vi "Main.vi"(11 "Module Admin":refnum<class "Delacor_lib_QMH_Module Admin.lvclass">) -> ()   [LabVIEW 2021, in "RT-TDMS-Logging.lvlib"]
doc: "This template is based off of the Queued Message Handler design pattern and the Queued Message Handler project template that ships with LabVIEW.\n\nThe main difference is that the queue is private to this module and communication between modules is performed via Broadcast and Request events.\n\nRequest events are wrapped in public API methods and are handled in the Event Handling Loop (EHL) of this VI. Any module can register for Broadcast events sent by this module. The EHL generates messages based on user interface actions.\n\nThe Message Handling Loop (MHL) processes messages generated by the EHL, or by other messages. The messages are string values, so new messages can be added easily to the Message Cases case structure in the MHL. Each message cluster can also provide an optional value for Message Data, which is a variant that can be converted to whatever message-specific data is required.\n_____\nBased on DQMH Project Template 7.0.1.1316."
uses:
  RT-TDMS-Logging.lvlib
  <vilib>/Delacor/Delacor QMH/Libraries/Module Admin_class/Delacor_lib_QMH_Module Admin.lvclass
  Module Data--cluster.ctl
  <vilib>/Wovalab/Utilities/Helper Loop Periodic Timing/Helper Loop Periodic Timing.lvclass/Helper Loop Periodic Timing.ctl
  <vilib>/Delacor/Delacor QMH/Libraries/Message Queue_class/Delacor_lib_QMH_Message Queue.lvclass/Delacor_lib_QMH_Message Queue.ctl
  Start Logging Argument--cluster.ctl
  Data Logging Duration Argument--cluster.ctl
  Stop Argument--cluster.ctl
  <vilib>/Delacor/Delacor QMH/Libraries/Module Admin_class/Delacor_lib_QMH_Module Admin.lvclass/Delacor_lib_QMH_Module Admin.ctl
  AI Data's Argument--cluster.ctl
  DO Data Argument--cluster.ctl
  <vilib>/Utility/miscctls.llb/LVPointTypeDef.ctl
  Main Engine/Controls/Main Engine Q Option.ctl
  Host-Control's/TCP Tx-Rx cluster.ctl
  <vilib>/Delacor/Delacor QMH/Libraries/Message Queue_class/Delacor_lib_QMH_Enqueue Message (Single).vi
  <vilib>/Delacor/Delacor QMH/Libraries/Module Admin_class/Delacor_lib_QMH_Get External Launch.vi
  <vilib>/Wovalab/Utilities/Helper Loop Periodic Timing/U32 Max Value--constant.vi
  <vilib>/Wovalab/Utilities/Helper Loop Periodic Timing/Update Last Execution Time.vi
  <vilib>/Wovalab/Utilities/Helper Loop Periodic Timing/Helper Loop Periodic Timing.lvclass
  <vilib>/Delacor/Delacor QMH/Libraries/Message Queue_class/Delacor_lib_QMH_Message Queue.lvclass
  <vilib>/addons/_JKI.lib/Serialization/JSON/JKI JSON Serialization.lvlib
panel:
  out "error out":errorcluster
  out "Status":string
  in  "Simulate MHL Error":bool
  in  "Simulate EHL Error":bool
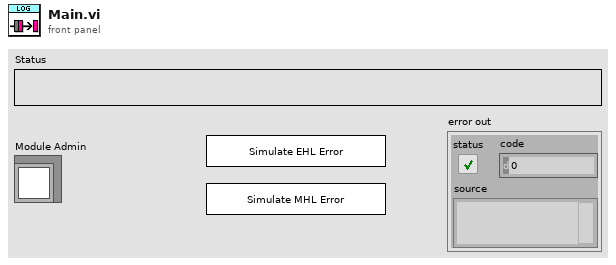
[diagram p1: front panel]
types:
  T1 = typedef "RT-TDMS-Logging.lvlib/Request Events--cluster.ctl" = cluster{"Stop Module":refnum<user-event>, "Show Panel":refnum<user-event>, "Hide Panel":refnum<user-event>, "Get Module Execution Status":refnum<user-event>, "Show Diagram":refnum<user-event>, "Data Logging Duration":refnum<user-event>, "AI Data's":refnum<user-event>, "Start Logging":refnum<user-event>, "DO Data":refnum<user-event>}
  T2 = typedef "RT-TDMS-Logging.lvlib/Start Logging Argument--cluster.ctl" = cluster{"Start Logging":variant}
  T3 = enum32{"invalid lock state", "Not Locked", "Locked (No Password)", "Password-protected"}
  T4 = typedef "RT-TDMS-Logging.lvlib/Stop Argument--cluster.ctl" = cluster{"Origin":string, "Exit via Stop Module Req?":bool, "Wait for Module to stop?":bool}
  T5 = typedef "RT-TDMS-Logging.lvlib/AI Data's Argument--cluster.ctl" = cluster{"AI Data's":variant}
  T6 = typedef "RT-TDMS-Logging.lvlib/DO Data Argument--cluster.ctl" = cluster{"DO Data":variant}
  T7 = typedef "LVPointTypeDef.ctl" = cluster{"Horizontal":i16, "Vertical":i16}
  T8 = enum32{"Invalid", "Standard", "Closed", "Hidden", "Minimized", "Maximized"}
  T9 = typedef "Main Engine Q Option.ctl" = enum16{"Init", "Get"}
  T10 = cluster{"Time Stamp":timestamp[], "Identification Names":string[], "Data":dbl[]}
  T11 = cluster{"Identification Name":string[], "Data":i16[]}
  T12 = enum16{"open", "open or create", "create or replace", "create", "open (read-only)"}
  T13 = typedef "TCP Tx-Rx cluster.ctl" = cluster{"Interface":string, "Command":string, "SubCmd":string, "Data":variant}
  T14 = typedef "RT-TDMS-Logging.lvlib/Module Data--cluster.ctl" = cluster{"Status":string, "TDMS-Folder":path, "Data Logging Time (S)":dbl, "Start -Log":bool, "Stop -Log":bool, "tdms file out":refnum<k34>, "Start Time":timestamp, "Interface Data's":cluster{"AO Data's":map{string, dbl}, "DI Data's":map{string, i16}, "DO Data's":map{string, i16}, "AI Data's":map{string, waveform(dbl)}}, "TCP Enigine Q":refnum<queue>}
  T15 = typedef "RT-TDMS-Logging.lvlib/Data Logging Duration Argument--cluster.ctl" = cluster{"Data Logging Duration(Sec)":dbl}
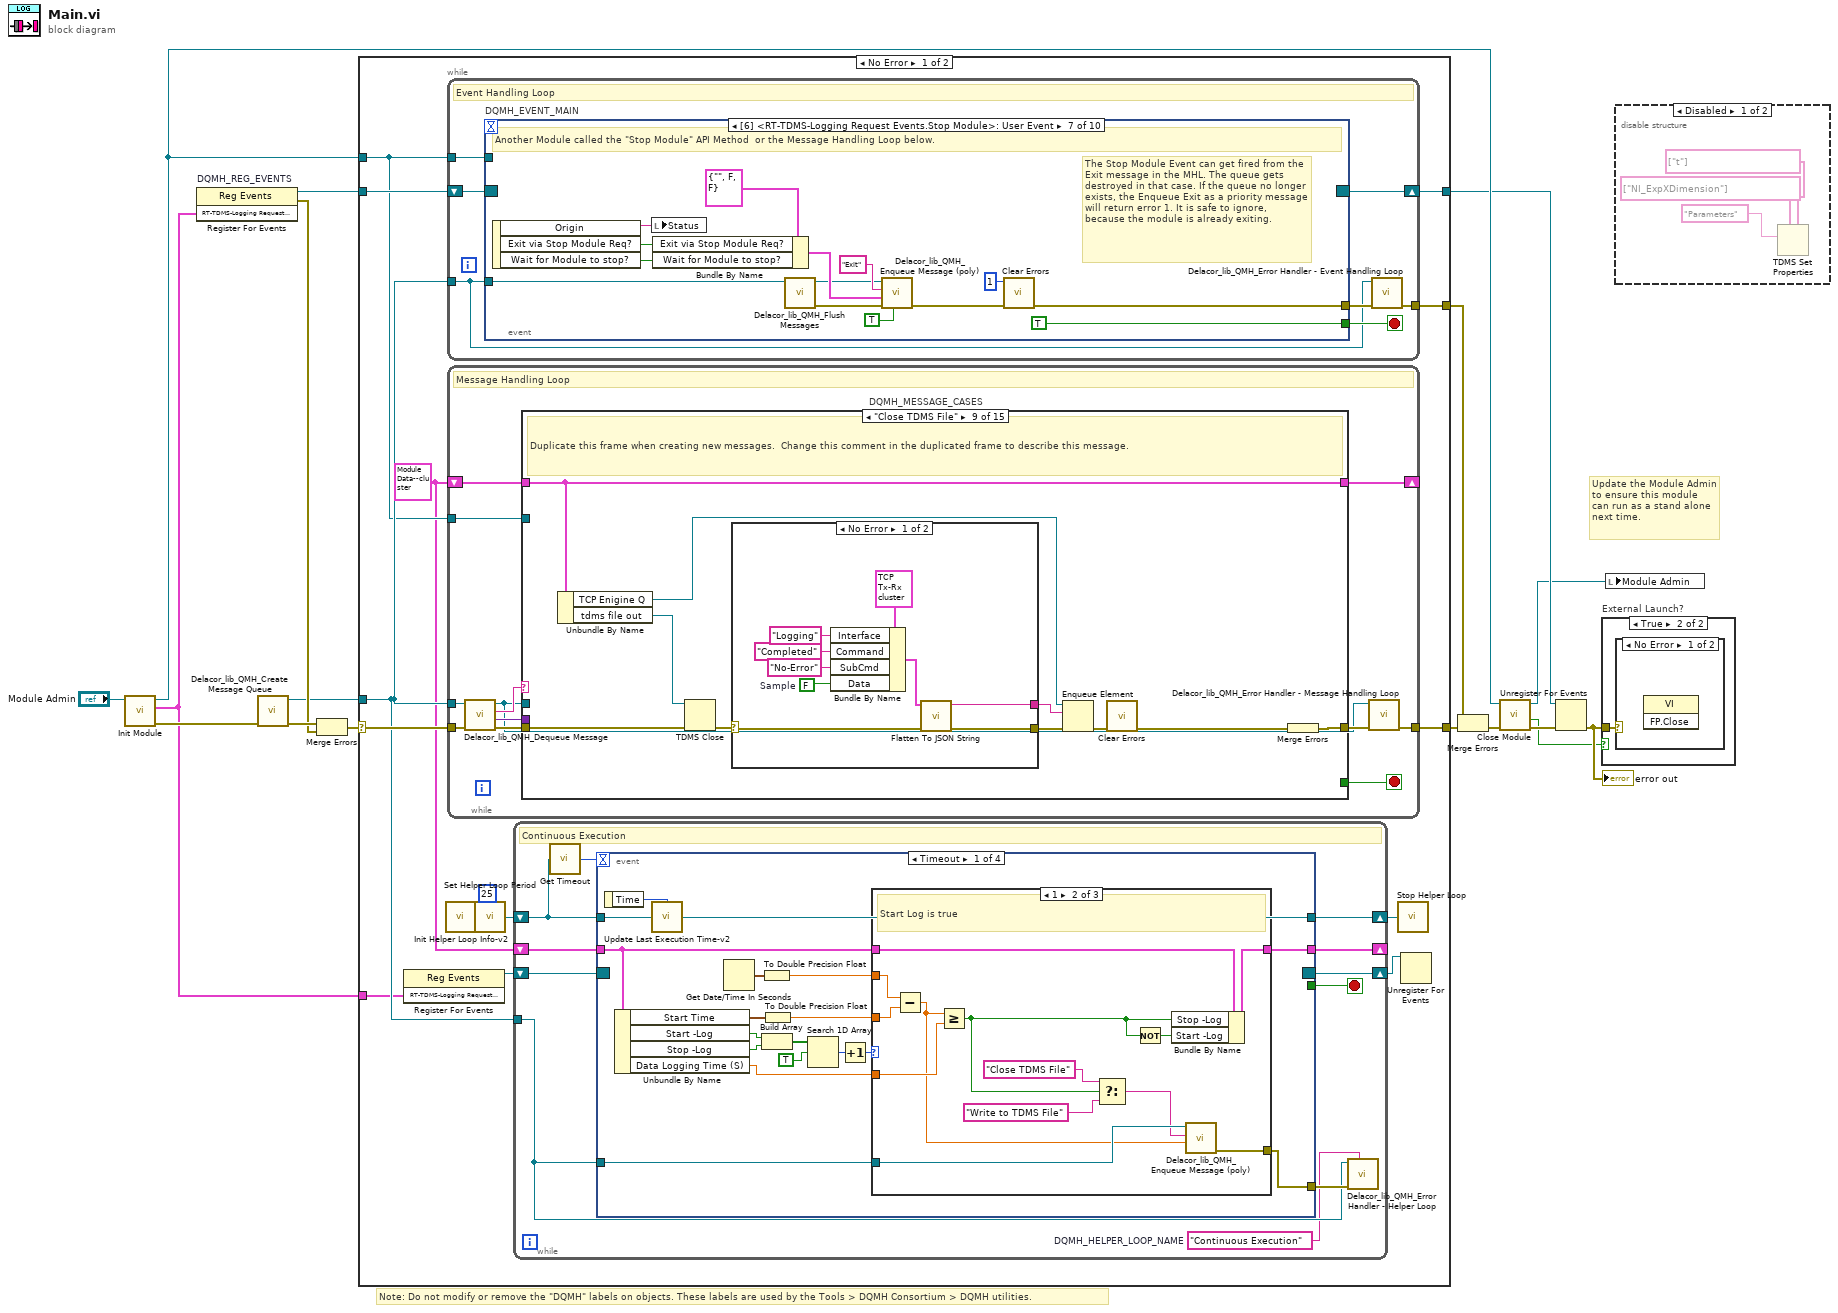
[diagram p0: block diagram]
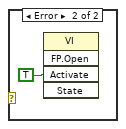
[diagram p4: hidden frame]
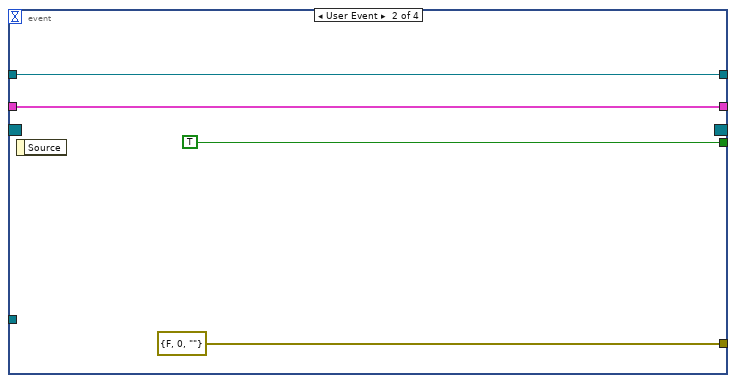
[diagram p7: hidden frame]
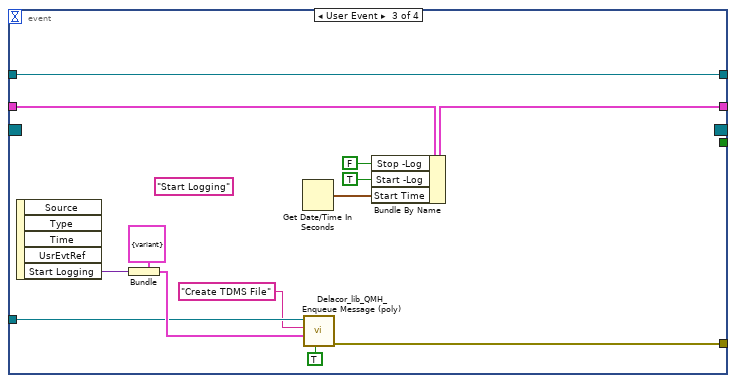
[diagram p8: hidden frame]
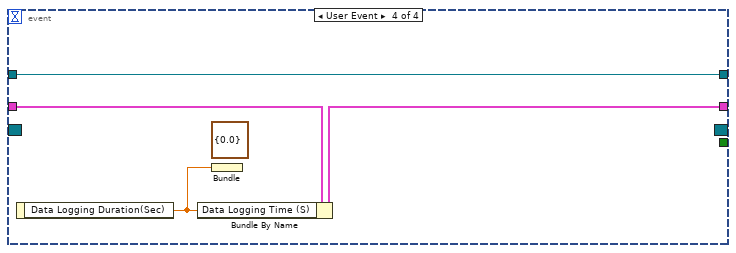
[diagram p9: hidden frame]
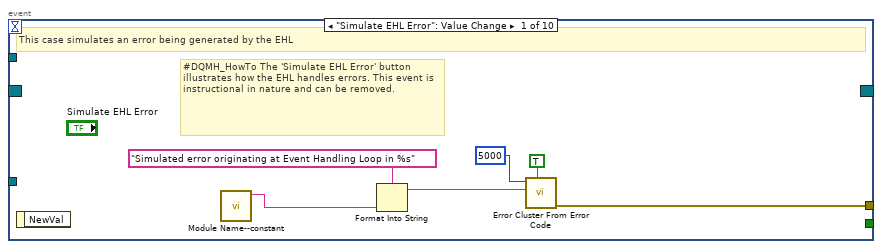
[diagram p10: hidden frame]
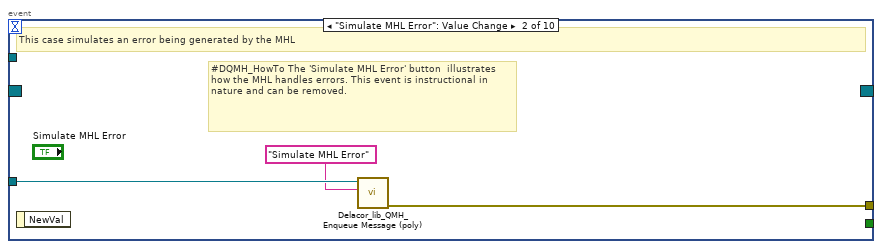
[diagram p11: hidden frame]
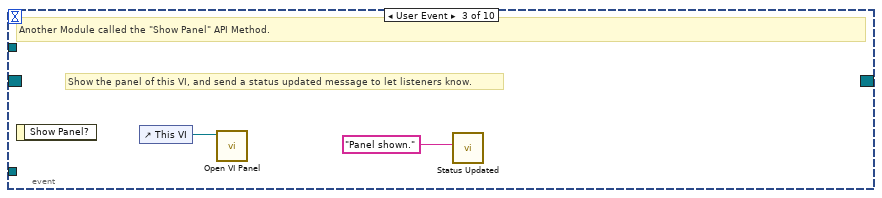
[diagram p12: hidden frame]
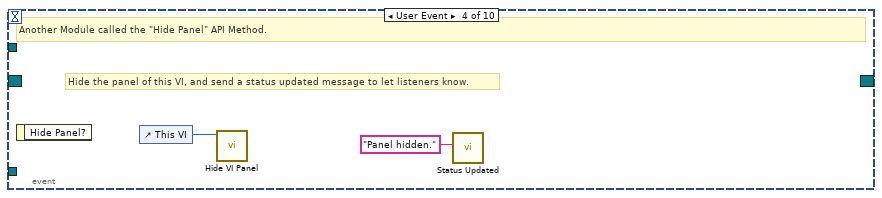
[diagram p13: hidden frame]
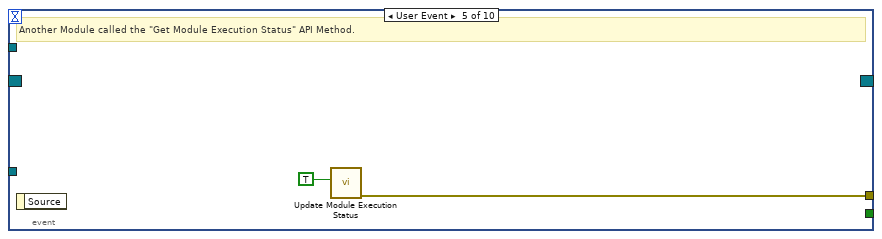
[diagram p14: hidden frame]
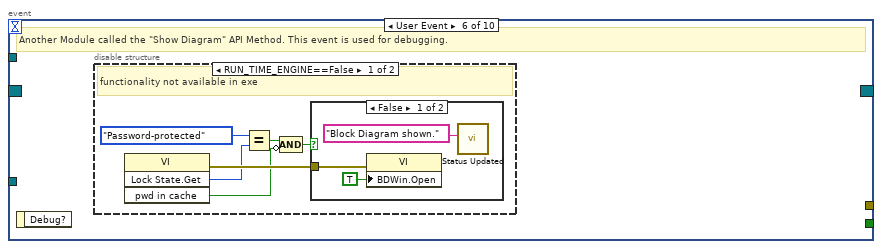
[diagram p15: hidden frame]
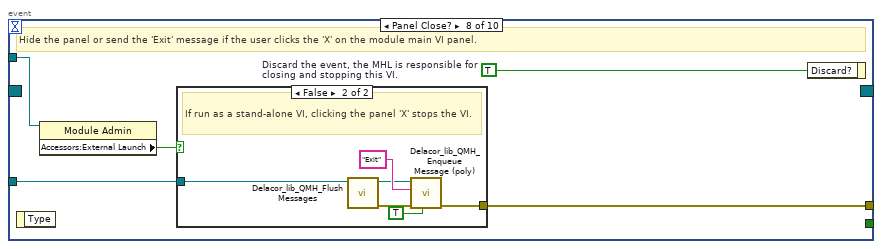
[diagram p18: hidden frame]
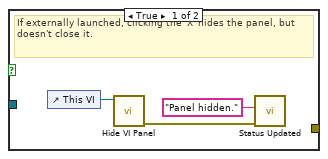
[diagram p19: hidden frame]
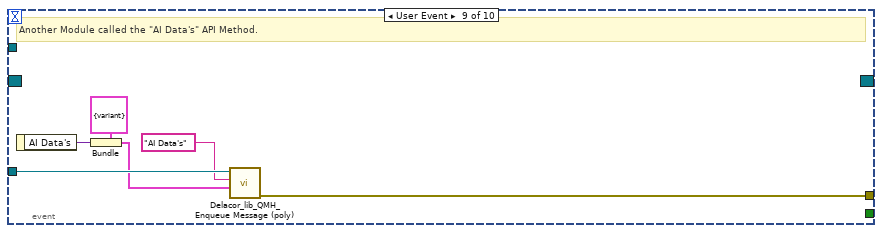
[diagram p20: hidden frame]
diagram:
  # "Note: Do not modify or remove the \"DQMH\" labels on objects. These labels are used by the Tools > DQMH Consortium > DQMH utilities."
  # "Update the Module Admin to ensure this module can run as a stand alone next time."
  n1 = call "Init Module.vi"("Singleton Module Admin in"="Module Admin") -> ("error out"=w16:errorcluster, "RT-TDMS-Logging Request Events"=w1:T1, "Singleton Module Admin out"=w8:refnum<class "Delacor_lib_QMH_Module Admin.lvclass">)  [unwired: 8 in]
  n2 = register-events "DQMH_REG_EVENTS"(w1) -> (reference out=w6:refnum<event-registration>, error out=w9:errorcluster)  [unwired: 2 in]
  n3 = call <vilib>:"Delacor_lib_QMH_Create Message Queue.vi"("error in"=w16) -> ("error out"=w11:errorcluster, "Message Queue"=w5:refnum<class "Delacor_lib_QMH_Message Queue.lvclass">)  [unwired: 9 in]
  n4 = Merge Errors(w11, w9) -> (w10:errorcluster)
  n5 = case shown="No Error" w10 {
    selector: w10 -> [w30 w438]
    tunnel: [w32 w437] -> w17
    tunnel: [w29 w436] -> w7
    tunnel: w6 -> [w28 w436]
    tunnel: w5 -> [w27 w431]
    tunnel: [w31 _] -> w14
    tunnel: w8 -> [w26 w432]
    tunnel: w1 -> [w25 _]
    frame No Error {
      w18 = T14 {"Status"="", "TDMS-Folder"=path "", "Data Logging Time (S)"=0.0, "Start -Log"=FALSE, "Stop -Log"=FALSE, "tdms file out"=refnum, "Start Time"=timestamp(0 s since 1904-01-01), "Interface Data's"={"AO Data's"={}, "DI Data's"={}, "DO Data's"={}, "AI Data's"={}}, "TCP Enigine Q"=refnum} ("Data Cluster")
      n6 = register-events ("DQMH_HELPER_REGFOREVENTS")(w25) -> (reference out=w23:refnum<event-registration>)  [unwired: 2 in, 1 out]
      n7 = call <vilib>:"Init Helper Loop Info-v2.vi"() -> ("Helper Loop Periodic Timing"=w21:refnum<class "Helper Loop Periodic Timing.lvclass">)  [unwired: 1 in]
      n8 = while {
        tunnel: w27 -> [w98]
        shift-right: [w101] -> w29
        shift-left: w28 -> [w102]
        tunnel: [w103] -> w31
        tunnel: w26 -> [w99]
        stop <- w100 stop-if-true
        # "Event Handling Loop"
        n9 = event "DQMH_EVENT_MAIN" shown="[6] <RT-TDMS-Logging Request Events.Stop Module>: User Event" {
          selector: w102 -> [_ _ _ _ _ _ _ _ _ _]
          dyn-events: [_ _ _ _ _ _ _ _ _ _] -> w101
          timeout: _ -> [_ _ _ _ _ _ _ _ _ _]
          tunnel: [_ _ _ _ _ _ TRUE ("Discard?") _ _ _] -> w100
          tunnel: w98 -> [_ w112 _ _ _ _ w131 w145 w162 w168]
          tunnel: [w110 w113 _ _ w119 _ w141 w147 w157 w163] -> w104
          tunnel: w99 -> [_ _ _ _ _ _ _ w144 _ _]
          event "Simulate EHL Error": Value Change {
            # "#DQMH_HowTo The 'Simulate EHL Error' button  illustrates how the EHL handles errors. This event is instructional in nature and can be removed."
            # "This case simulates an error being generated by the EHL"
            n10 = event-data() -> ()  [unwired: 1 in, 1 out]
            n11 = call "Module Name--constant.vi"() -> ("Module Name"=w107:string)  [unwired: 11 in]
            n12 = Format Into String(format string="Simulated error originating at Event Handling Loop in %s", w107) -> (resulting string=w108:string)  [unwired: 2 in, 1 out]
            n13 = call <vilib>:"Error Cluster From Error Code.vi"("show call chain? (False)"=TRUE, "error message (\"\")"=w108, "error code (0)"=5000) -> ("error out"=w110:errorcluster)  [unwired: 6 in]
          }
          event "Simulate MHL Error": Value Change {
            # "#DQMH_HowTo The 'Simulate MHL Error' button  illustrates how the MHL handles errors. This event is instructional in nature and can be removed."
            # "This case simulates an error being generated by the MHL"
            n14 = event-data() -> ()  [unwired: 1 in, 1 out]
            n15 = call-poly <vilib>:"Delacor_lib_QMH_Enqueue Message (poly).vi"("Message"="Simulate MHL Error", "Message Queue in"=w112) -> ("error out"=w113:errorcluster)  [unwired: 8 in, 1 out]
          }
          event User Event {
            # "Show the panel of this VI, and send a status updated message to let listeners know."
            # "Another Module called the \"Show Panel\" API Method."
            n16 = event-data() -> ()  [unwired: 1 in, 1 out]
            n17 = control-ref of="This VI"() -> (w115:refnum<vi>)
            n18 = call "Open VI Panel.vi"("VI"=w115) -> ()  [unwired: 10 in, 1 out]
            n19 = call "Status Updated.vi"("Status"="Panel shown." ("format string")) -> ()  [unwired: 10 in, 1 out]
          }
          event User Event {
            # "Hide the panel of this VI, and send a status updated message to let listeners know."
            # "Another Module called the \"Hide Panel\" API Method."
            n20 = event-data() -> ()  [unwired: 1 in, 1 out]
            n21 = control-ref of="This VI"() -> (w117:refnum<vi>)
            n22 = call "Hide VI Panel.vi"("VI"=w117) -> ()  [unwired: 10 in, 1 out]
            n23 = call "Status Updated.vi"("Status"="Panel hidden." ("format string")) -> ()  [unwired: 10 in, 1 out]
          }
          event User Event {
            # "Another Module called the \"Get Module Execution Status\" API Method."
            n24 = event-data() -> ()  [unwired: 1 in, 1 out]
            n25 = call "Update Module Execution Status.vi"("Running?"=TRUE) -> ("error out"=w119:errorcluster)  [unwired: 10 in]
          }
          event User Event {
            # "Another Module called the \"Show Diagram\" API Method. This event is used for debugging."
            n26 = event-data() -> ()  [unwired: 1 in, 1 out]
            n27 = disable-structure shown="RUN_TIME_ENGINE==False" {
              frame condition #0 (active) {
                # "functionality not available in exe"
                n28 = invoke on="Invoke Node" class="VI" method="Lock State.Get"() -> (error out=w125:errorcluster, "Get Lock State"=w124:T3, "pwd in cache"=w121:bool)  [unwired: 4 in, 1 out]
                n29 = Equal?(x=T3."Password-protected", y=w124) -> (x = y?=w122:bool)
                n30 = Compound Arithmetic op=AND(w122, invert w121) -> (w120:bool)
                n31 = case shown="False" w120 {
                  tunnel: w125 -> [w128 _]
                  frame False {
                    n32 = property on="Property Node" class="VI"(error in=w128, "BDWin.Open"=TRUE ("Block Diagram Window:Open")) -> ()  [unwired: 1 in, 2 out]
                    n33 = call "Status Updated.vi"("Status"="Block Diagram shown." ("format string")) -> ()  [unwired: 10 in, 1 out]
                  }
                  frame True {
                    # "Password-protected VI, and the password is not in the cache. Do not show the diagram."
                  }
                }
              }
              frame condition #1 {
              }
            }
          }
          event User Event {
            # "The Stop Module Event can get fired from the Exit message in the MHL. The queue gets destroyed in that case. If the queue no longer exists, the Enqueue Exit as a priority message will return error 1. It is safe to ignore, because the module is already exiting."
            # "Another Module called the \"Stop Module\" API Method  or the Message Handling Loop below."
            n34 = event-data() -> ("Origin"=w138:string, "Exit via Stop Module Req?"=w134:bool, "Wait for Module to stop?"=w133:bool)  [unwired: 1 in]
            n35 = local write "Status"(w138) -> ()
            n36 = Bundle By Name(cluster=T4 {"Origin"="", "Exit via Stop Module Req?"=FALSE, "Wait for Module to stop?"=FALSE} ("Stop Argument"), "Exit via Stop Module Req?"=w134, "Wait for Module to stop?"=w133) -> (w132:T4)
            n37 = call-dynamic "Delacor_lib_QMH_Flush Messages.vi"("Message Queue in"=w131) -> ("error out"=w129:errorcluster, "Message Queue out"=w130:refnum<class "Delacor_lib_QMH_Message Queue.lvclass">)  [unwired: 7 in, 2 out]
            n38 = call-poly <vilib>:"Delacor_lib_QMH_Enqueue Message (poly).vi"("Priority Message? (F)"=TRUE, "error in"=w129, "Message Data"=w132, "Message"="Exit", "Message Queue in"=w130) -> ("error out"=w142:errorcluster)  [unwired: 5 in, 1 out]
            n39 = call <vilib>:"Clear Errors.vi"("error in (no error)"=w142, "specific error code to clear (0: all)"=1) -> ("error out"=w141:errorcluster)  [unwired: 4 in, 1 out]
          }
          event Panel Close? {
            w146 = TRUE  # Discard the event, the MHL is responsible for closing and stopping this VI.
            # "Hide the panel or send the 'Exit' message if the user clicks the 'X' on the module main VI panel."
            n40 = event-data() -> ()  [unwired: 1 in, 1 out]
            n41 = property on="Property Node" class="Module Admin"(reference=w144) -> ("Accessors:External Launch"=w143:bool)  [unwired: 1 in, 2 out]
            n42 = case shown="False" w143 {
              tunnel: w145 -> [_ w153]
              tunnel: [_ w156] -> w147
              frame True {
                # "If externally launched, clicking the 'X' hides the panel, but doesn't close it."
                n43 = control-ref of="This VI"() -> (w150:refnum<vi>)
                n44 = call "Hide VI Panel.vi"("VI"=w150) -> ("error out"=w148:errorcluster)  [unwired: 10 in]
                n45 = call "Status Updated.vi"("error in"=w148, "Status"="Panel hidden." ("format string")) -> ()  [unwired: 9 in, 1 out]
              }
              frame False {
                # "If run as a stand-alone VI, clicking the panel 'X' stops the VI."
                n46 = call-dynamic "Delacor_lib_QMH_Flush Messages.vi"("Message Queue in"=w153) -> ("error out"=w151:errorcluster, "Message Queue out"=w152:refnum<class "Delacor_lib_QMH_Message Queue.lvclass">)  [unwired: 7 in, 2 out]
                n47 = call-poly <vilib>:"Delacor_lib_QMH_Enqueue Message (poly).vi"("Priority Message? (F)"=TRUE, "error in"=w151, "Message"="Exit", "Message Queue in"=w152) -> ("error out"=w156:errorcluster)  [unwired: 6 in, 1 out]
              }
            }
            n48 = event-data ("Event Filter Node")("Discard?"=w146) -> ()  [unwired: 1 in, 1 out]
          }
          event User Event {
            # "Another Module called the \"AI Data's\" API Method."
            n49 = event-data() -> ("AI Data's"=w158:variant)  [unwired: 1 in]
            n50 = Bundle(cluster=T5 {"AI Data's"=variant} ("AI Data's Argument"), "AI Data's"=w158) -> (w159:T5)
            n51 = call-poly <vilib>:"Delacor_lib_QMH_Enqueue Message (poly).vi"("Message Data"=w159, "Message"="AI Data's", "Message Queue in"=w162) -> ("error out"=w157:errorcluster)  [unwired: 7 in, 1 out]
          }
          event User Event {
            # "Another Module called the \"DO Data\" API Method."
            n52 = event-data() -> ("DO Data"=w164:variant)  [unwired: 1 in]
            n53 = Bundle(cluster=T6 {"DO Data"=variant} ("DO Data Argument"), "DO Data"=w164) -> (w165:T6)
            n54 = call-poly <vilib>:"Delacor_lib_QMH_Enqueue Message (poly).vi"("Message Data"=w165, "Message"="DO Data", "Message Queue in"=w168) -> ("error out"=w163:errorcluster)  [unwired: 7 in, 1 out]
          }
        }
        n55 = call-dynamic "Delacor_lib_QMH_Error Handler - Event Handling Loop.vi"("error in"=w104, "Message Queue in"=w98) -> ("dup error in"=w103:errorcluster)  [unwired: 8 in, 1 out]
      }
      n56 = while {
        tunnel: w27 -> [w169]
        shift-right: [w177] -> _
        shift-left: w18 -> [w178]
        tunnel: w30 -> [w180]
        tunnel: [w172] -> w32
        tunnel: w26 -> [w173]
        stop <- w176 stop-if-true
        # "Message Handling Loop"
        n57 = call-dynamic "Delacor_lib_QMH_Dequeue Message.vi"("error in"=w180, "Message Queue in"=w169) -> ("error out"=w179:errorcluster, "Message Data"=w174:variant, "Message"=w175:string, "Message Queue out"=w170:refnum<class "Delacor_lib_QMH_Message Queue.lvclass">)  [unwired: 6 in]
        n58 = case "DQMH_MESSAGE_CASES" shown="\"Close TDMS File\"" w175 {
          selector: w175 -> [_ _ _ _ _ _ _ _ _ _ _ _ _ _ w426]
          tunnel: w170 -> [w181 _ _ _ _ _ _ _ _ _ _ _ w392 w414 _]
          tunnel: w179 -> [w202 w209 w227 w237 w275 w301 w318 w341 w353 w377 w379 w388 w399 w420 w429]
          tunnel: [w182 w210 w227 w231 w269 w301 w320 w346 w356 w376 w379 w387 w395 w415 w430] -> w171
          tunnel: w178 -> [w192 w207 w226 w229 w268 w300 w310 w344 w355 w375 w378 w385 w394 w413 w427]
          tunnel: [w191 w205 w226 w228 w267 w300 w309 w343 w355 w375 w378 w385 w394 w413 w427] -> w177
          tunnel: [_ _ _ _ _ _ _ _ _ _ _ _ _ w412 _] -> w176
          tunnel: w174 -> [_ _ _ w236 w274 _ _ w342 _ _ _ _ w393 w411 _]
          tunnel: w173 -> [w193 _ _ _ _ _ _ _ _ _ _ _ w391 w406 _]
          frame "Initialize" {
            w187 = "Initial Message" ("Initial Message")
            # "Initialize - Any operation that needs to be done before the module can receive messages. Synchronize Caller Events.vi will inform Start Module.vi that the module has launched and is ready to receive messages. Module Did Init.vi will broadcast that the module initialized."
            n59 = call "Synchronize Caller Events.vi"("error in"=w202, "Singleton Module Admin in"=w193) -> ("error out"=w201:errorcluster, "Singleton Module Admin out"=w188:refnum<class "Delacor_lib_QMH_Module Admin.lvclass">)  [unwired: 8 in]
            n60 = property on="Property Node" class="Module Admin"(reference=w188) -> ("Accessors:External Launch"=w197:bool)  [unwired: 1 in, 2 out]
            n61 = Select(t=T8."Closed" ("State"), s=w197, f=T8."Closed" ("State")) -> (s? t:f=w194:T8)
            n62 = call "Module Name--constant.vi"() -> ("Module Name"=w200:string)  [unwired: 11 in]
            n63 = property on="Property Node" class="VI"("Front Panel.Title"=w200) -> (reference out=w199:refnum<vi>, error out=w204:errorcluster)  [unwired: 2 in]
            n64 = call "Module Name--constant.vi"() -> ("Module Name"=w189:string)  [unwired: 11 in]
            n65 = invoke on="Invoke Node" class="VI" method="FP.Open"(reference=w199, error in=w204, "State"=w194) -> (reference out=w198:refnum<vi>, error out=w203:errorcluster)  [unwired: 2 in, 3 out]
            n66 = Bundle By Name(cluster=w192, "Status"=w187) -> (w191:T14)
            n67 = call "Module Did Init.vi"("error in"=w201, "Initialized?"=TRUE, "Origin"=w189) -> ("error out"=w183:errorcluster)  [unwired: 8 in]
            n68 = invoke on="Invoke Node" class="VI" method="FP.Center"(reference=w198, error in=w203) -> (error out=w185:errorcluster)  [unwired: 1 in, 2 out]
            n69 = call <vilib>:"Clear Errors.vi"("error in (no error)"=w185) -> ()  [unwired: 5 in, 2 out]
            n70 = property on="Pane" class="Pane"("Origin"=T7 {"Horizontal"=0, "Vertical"=0}) -> ()  [unwired: 2 in, 2 out]
            n71 = call-poly <vilib>:"Delacor_lib_QMH_Enqueue Message (poly).vi"("error in"=w183, "Message"="Init-1", "Message Queue in"=w181) -> ("error out"=w182:errorcluster)  [unwired: 7 in, 1 out]
            "Status" <- w187
          }
          frame "Init-1" {
            # "Duplicate this frame when creating new messages.  Change this comment in the duplicated frame to describe this message."
            n72 = for {
              N: 11 -> [_]
              shift-right: [w215] -> w206
              shift-left: w209 -> [w214]
              shift-right: [w211] -> w205
              shift-left: w207 -> [w212]
              i -> [w213]
              n73 = case shown="0, Default" w213 {
                tunnel: [w218 w225] -> w215
                tunnel: w214 -> [w222 w225]
                tunnel: w212 -> [w220 w224]
                tunnel: [w216 w224] -> w211
                frame 0, Default {
                  n74 = call "Main Engine & TCP Engine Q Init LV2GBL.vi"("Q Option"=Main_Engine_Q_Option."Get", "error in"=w222) -> ("error out"=w219:errorcluster, "TCP Enigine Tx-Q"=w217:refnum<queue>)  [unwired: 7 in, 1 out]
                  n75 = call "Main Engine Path and Folder Info.vi"("error in"=w219) -> ("error out"=w218:errorcluster, "TDMS-Logging"=w221:path)  [unwired: 4 in, 5 out]
                  n76 = Bundle By Name(cluster=w220, "TCP Enigine Q"=w217, "TDMS-Folder"=w221) -> (w216:T14)
                }
                frame 1 {
                }
              }
            }
            n77 = Merge Errors(w206) -> (w210:errorcluster)
          }
          frame "---Module Specific---" {
            # "Separator -- The following cases handle messages specific to this Module."
          }
          frame "AI Data's" {
            # "This Event will give the acquired data's from Analog Input Engine to the TDMS logging module."
            n78 = Variant To Data(error in=w237, type=T5 {"AI Data's"=variant} ("AI Data's Argument"), Variant=w236) -> (data=w234:T5, error out=w232:errorcluster)
            n79 = Unbundle By Name(w234) -> ("AI Data's"=w233:variant)
            n80 = in-place {
              in-place-border: w233 -> [w248]
              in-place-border: w232 -> [w247]
              in-place-border: [w244] -> w230
              n81 = in-place-cluster #1(w229) -> ("Interface Data's.AI Data's"=w241:map{string, waveform(dbl)})
              n82 = Variant To Data(error in=w247, type=T10 {"Time Stamp"=[], "Identification Names"=[], "Data"=[]} ("output cluster"), Variant=w248) -> (data=w246:T10, error out=w245:errorcluster)
              n83 = Unbundle By Name(w246) -> ("Identification Names"=w243:string[], "Data"=w242:dbl[], "Time Stamp"=w238:timestamp[])
              n84 = for {
                shift-right: [w251] -> w244
                shift-left: w245 -> [w250]
                tunnel: w243 -> [w253] mode=indexing
                tunnel: w242 -> [w254] mode=indexing
                shift-right: [w255] -> w240
                shift-left: w241 -> [w256]
                tunnel: w238 -> [w249] mode=indexing
                n85 = Empty String/Path?(string/path=w253) -> (empty?=w252:bool)
                n86 = case shown="False" w252 {
                  tunnel: w256 -> [w264 w266]
                  tunnel: [w263 w266] -> w255
                  tunnel: w254 -> [w260 _]
                  tunnel: w253 -> [w262 _]
                  tunnel: [w261 w265] -> w251
                  tunnel: w250 -> [w261 w265]
                  tunnel: w249 -> [w258 _]
                  frame False {
                    n87 = Build Array(w260) -> (w259:dbl[])
                    n88 = Bundle By Name("Y"=w259, "t0"=w258) -> (w257:waveform(dbl))  [unwired: 1 in]
                    n89 = Insert Into Map(map in=w264, key=w262, value=w257) -> (map out=w263:map{string, waveform(dbl)})  [unwired: 2 out]
                  }
                  frame True {
                  }
                }
              }
              n90 = in-place-cluster #1("Interface Data's.AI Data's"=w240) -> (w228:T14)
            }
            n91 = Merge Errors(w230) -> (w231:errorcluster)
          }
          frame "DO Data" {
            # "This event will receive the Digital Output Data which we need to Log."
            n92 = Variant To Data(error in=w275, type=T6 {"DO Data"=variant} ("DO Data Argument"), Variant=w274) -> (data=w272:T6, error out=w270:errorcluster)
            n93 = Unbundle By Name(w272) -> ("DO Data"=w271:variant)
            n94 = in-place {
              in-place-border: w271 -> [w285]
              in-place-border: w270 -> [w284]
              in-place-border: [w281] -> w269
              n95 = in-place-cluster #2(w268) -> ("Interface Data's.DO Data's"=w276:map{string, i16})
              n96 = Variant To Data(error in=w284, type=T11 {"Identification Name"=[], "Data"=[]} ("output cluster"), Variant=w285) -> (data=w282:T11, error out=w280:errorcluster)
              n97 = Unbundle By Name(w282) -> ("Identification Name"=w279:string[], "Data"=w278:i16[])
              n98 = for {
                shift-right: [w287] -> w281
                shift-left: w280 -> [w286]
                tunnel: w279 -> [w289] mode=indexing
                tunnel: w278 -> [w290] mode=indexing
                shift-right: [w291] -> w277
                shift-left: w276 -> [w292]
                n99 = Empty String/Path?(string/path=w289) -> (empty?=w288:bool)
                n100 = case shown="False" w288 {
                  tunnel: w292 -> [w297 w299]
                  tunnel: [w296 w299] -> w291
                  tunnel: w290 -> [w295 _]
                  tunnel: w289 -> [w294 _]
                  tunnel: [w293 w298] -> w287
                  tunnel: w286 -> [w293 w298]
                  frame False {
                    n101 = Insert Into Map(map in=w297, key=w294, value=w295) -> (map out=w296:map{string, i16})  [unwired: 2 out]
                  }
                  frame True {
                  }
                }
              }
              n102 = in-place-cluster #2("Interface Data's.DO Data's"=w277) -> (w267:T14)
            }
          }
          frame "-----File Operation's-----" {
            # "Separator -- The following cases handle messages specific to this Module."
          }
          frame "Create TDMS File" {
            # "Duplicate this frame when creating new messages.  Change this comment in the duplicated frame to describe this message."
            n103 = Unbundle By Name(w310) -> ("TCP Enigine Q"=w308:refnum<queue>, "TDMS-Folder"=w312:path)
            n104 = Get Date/Time In Seconds() -> (seconds since 1Jan1904=w317:timestamp)
            n105 = Format Date/Time String(time format string (%c)="%Y_%m_%d_%H_%M_%S", seconds (now)=w317) -> (date/time string=w315:string)  [unwired: 1 in]
            n106 = Concatenate Strings(w315, ".tdms" ("string")) -> (w313:string)
            n107 = Build Path(base path=w312, name or relative path=w313) -> (appended path=w311:path)
            n108 = TDMS Open(8:w318, 10:T12."open or create" ("operation (0:open)"), 11:w311) -> (0:w305:errorcluster, 3:w304:refnum<k34>)  [unwired: 4 in]
            n109 = Bundle By Name(cluster=w310, "tdms file out"=w304) -> (w309:T14)
            n110 = case shown="No Error" w305 {
              selector: w305 -> [w321 w330]
              tunnel: [w323 w331] -> w307
              tunnel: [w322 w332] -> w306
              tunnel: [w321 _] -> w302
              frame No Error {
                w324 = FALSE  # Sample
                n111 = Bundle By Name(cluster=T13 {"Interface"="CPU", "Command"="CPU Info", "SubCmd"="Monitor", "Data"=variant} ("TCP Tx-Rx Cluster"), "Interface"="Logging", "Command"="Started", "SubCmd"="No-Error" ("Interface Data.SubCmd"), "Data"=w324) -> (w326:T13)
                n112 = call <vilib>:"Flatten To JSON String.vi"("error in"=w321, "Variant"=w326) -> ("error out"=w322:errorcluster, "JSON String"=w323:string)  [unwired: 8 in]
              }
              frame Error {
                n113 = Bundle By Name(cluster=T13 {"Interface"="CPU", "Command"="CPU Info", "SubCmd"="Monitor", "Data"=variant} ("TCP Tx-Rx Cluster"), "Interface"="Logging", "Command"="Started", "SubCmd"="Error" ("Interface Data.SubCmd"), "Data"=w330) -> (w334:T13)
                n114 = call <vilib>:"Flatten To JSON String.vi"("Variant"=w334) -> ("error out"=w332:errorcluster, "JSON String"=w331:string)  [unwired: 9 in]
              }
            }
            n115 = Enqueue Element(queue=w308, element=w307, error in (no error)=w306) -> (error out=w303:errorcluster)  [unwired: 1 in, 2 out]
            n116 = call <vilib>:"Clear Errors.vi"("error in (no error)"=w303) -> ()  [unwired: 5 in, 2 out]
            n117 = Merge Errors(w302) -> (w320:errorcluster)
          }
          frame "Write to TDMS File" {
            # "Duplicate this frame when creating new messages.  Change this comment in the duplicated frame to describe this message."
            n118 = Variant To Data(error in=w341, type=0.0, Variant=w342) -> (data=w338:dbl, error out=w340:errorcluster)
            n119 = call "Write To TDMS File.vi"("Data Cluster In"=w344, "error in (no error)"=w340, "Releative Time"=w338) -> ("error out"=w345:errorcluster, "Data Cluster Out"=w343:T14)  [unwired: 7 in]
            n120 = Merge Errors(w345) -> (w346:errorcluster)
          }
          frame "Close TDMS File" {
            # "Duplicate this frame when creating new messages.  Change this comment in the duplicated frame to describe this message."
            n121 = Unbundle By Name(w355) -> ("TCP Enigine Q"=w351:refnum<queue>, "tdms file out"=w354:refnum<k34>)
            n122 = TDMS Close(8:w353, 11:w354) -> (0:w352:errorcluster)  [unwired: 1 out]
            n123 = case shown="No Error" w352 {
              selector: w352 -> [w359 w366]
              tunnel: [w358 w368] -> w350
              tunnel: [w357 w369] -> w349
              frame No Error {
                w360 = FALSE  # Sample
                n124 = Bundle By Name(cluster=T13 {"Interface"="CPU", "Command"="CPU Info", "SubCmd"="Monitor", "Data"=variant} ("TCP Tx-Rx Cluster"), "Interface"="Logging", "Command"="Completed", "SubCmd"="No-Error" ("Interface Data.SubCmd"), "Data"=w360) -> (w362:T13)
                n125 = call <vilib>:"Flatten To JSON String.vi"("error in"=w359, "Variant"=w362) -> ("error out"=w357:errorcluster, "JSON String"=w358:string)  [unwired: 8 in]
              }
              frame Error {
                n126 = Bundle By Name(cluster=T13 {"Interface"="CPU", "Command"="CPU Info", "SubCmd"="Monitor", "Data"=variant} ("TCP Tx-Rx Cluster"), "Interface"="Logging", "Command"="Completed", "SubCmd"="Error" ("Interface Data.SubCmd"), "Data"=w366) -> (w371:T13)
                n127 = call <vilib>:"Clear Errors.vi"("error in (no error)"=w366) -> ("error out"=w367:errorcluster)  [unwired: 5 in, 1 out]
                n128 = call <vilib>:"Flatten To JSON String.vi"("error in"=w367, "Variant"=w371) -> ("error out"=w369:errorcluster, "JSON String"=w368:string)  [unwired: 8 in]
              }
            }
            n129 = Enqueue Element(queue=w351, element=w350, error in (no error)=w349) -> (error out=w348:errorcluster)  [unwired: 1 in, 2 out]
            n130 = call <vilib>:"Clear Errors.vi"("error in (no error)"=w348) -> ("error out"=w347:errorcluster)  [unwired: 5 in, 1 out]
            n131 = Merge Errors(w347) -> (w356:errorcluster)
          }
          frame "---Copy This Frame---" {
            # "Duplicate this frame when creating new messages.  Change this comment in the duplicated frame to describe this message."
            n132 = Merge Errors(w377) -> (w376:errorcluster)
          }
          frame "---Exit and Error Handling---" {
            # "Separator - The following cases handle errors and exit messages."
          }
          frame "Simulate MHL Error" {
            # "#DQMH_HowTo The 'Simulate MHL Error' button  illustrates how the MHL handles errors. This event is instructional in nature and can be removed."
            # "Simulate an error occurring at the MHL"
            n133 = call "Module Name--constant.vi"() -> ("Module Name"=w381:string)  [unwired: 11 in]
            n134 = Format Into String(format string="Simulated error originating at Message Handling Loop in %s", w381) -> (resulting string=w382:string)  [unwired: 2 in, 1 out]
            n135 = call <vilib>:"Error Cluster From Error Code.vi"("show call chain? (False)"=TRUE, "error message (\"\")"=w382, "error code (0)"=5001) -> ("error out"=w386:errorcluster)  [unwired: 6 in]
            n136 = Merge Errors(w388, w386) -> (w387:errorcluster)
          }
          frame "Error" {
            # "Error - Check the error message data and respond accordingly. This message is sent by the \"Error Handler\" VIs at the end of each loop in this application."
            n137 = property on="Property Node" class="Module Admin"(reference=w391) -> ("Accessors:External Launch"=w390:bool)  [unwired: 1 in, 2 out]
            n138 = Variant To Data(error in=w399, type=errorcluster {"status"=FALSE, "code"=0, "source"=""} ("error constant"), Variant=w393) -> (data=w389:errorcluster, error out=w397:errorcluster)
            n139 = local write "error out"(w389) -> ()
            n140 = call "Error Reported.vi"("Error"=w389) -> ()  [unwired: 10 in, 1 out]
            n141 = case shown="True" w390 {
              tunnel: [w404 _] -> w396
              tunnel: w392 -> [w402 _]
              tunnel: w389 -> [w403 _]
              frame False {
                n142 = disable-structure shown="DQMH_Disable_SEH==TRUE" {
                  disable-tunnel: w403 -> [w405 _]
                  frame condition #0 (active) {
                    # "If the module is running standalone, then pop up an error dialog and call the \"Exit\" message."
                    n143 = call <vilib>:"Simple Error Handler.vi"("error in (no error)"=w405) -> ()  [unwired: 4 in, 5 out]
                  }
                  frame condition #1 {
                    # "To prevent the Simple Error Handler VI from being loaded (e.g. when deploying to a Real-Time target), add the Conditional Disable Symbol \"DQMH_Disable_SEH\" to your project and set it to TRUE."
                  }
                }
                n144 = call-poly <vilib>:"Delacor_lib_QMH_Enqueue Message (poly).vi"("Priority Message? (F)"=TRUE, "Message"="Exit", "Message Queue in"=w402) -> ("error out"=w404:errorcluster)  [unwired: 7 in, 1 out]
              }
              frame True {
                # "If the module was launched externally, calling the Error Reported broadcast VI is the only action performed by the \"Error\" message. The module's caller can then process the error appropriately."
              }
            }
            n145 = Merge Errors(w397, w396) -> (w395:errorcluster)
          }
          frame "Exit" {
            w410 = 91  # 91: not all Exit messages will have an argument
            w412 = TRUE  # Stop the VI
            # "Release the message queue reference"
            # "Exit - Exit the application."
            n146 = Variant To Data(error in=w420, type=T4 {"Origin"="", "Exit via Stop Module Req?"=FALSE, "Wait for Module to stop?"=FALSE} ("Stop Argument"), Variant=w411) -> (data=w408:T4, error out=w417:errorcluster)
            n147 = call <vilib>:"Clear Errors.vi"("error in (no error)"=w417, "specific error code to clear (0: all)"=w410) -> ("error out"=w419:errorcluster)  [unwired: 4 in, 1 out]
            n148 = control-ref of="This VI"() -> (w407:refnum<vi>)
            n149 = call-dynamic "Delacor_lib_QMH_Release Message Queue.vi"("error in"=w419, "Message Queue"=w414) -> ("error out"=w418:errorcluster)  [unwired: 9 in]
            n150 = call "Handle Exit.vi"("Stop Argument"=w408, "Admin in"=w406, "VI reference"=w407) -> ("error out"=w416:errorcluster)  [unwired: 7 in, 1 out]
            n151 = Merge Errors(w418, w416) -> (w415:errorcluster)
            n152 = call "Error Reported.vi"("Error"=w415) -> ()  [unwired: 10 in, 1 out]
          }
          frame Default {
            # "'Default' case only runs if there is a message that isn't defined in any of the other cases.  Output a programming error."
            n153 = call "Module Name--constant.vi"() -> ("Module Name"=w425:string)  [unwired: 11 in]
            n154 = Format Into String(format string="The invalid message string \"%s\" was received in the Message Handling Loop for module \"%s\".", w426, w425) -> (resulting string=w421:string)  [unwired: 2 in, 1 out]
            n155 = call <vilib>:"Error Cluster From Error Code.vi"("show call chain? (False)"=TRUE, "error message (\"\")"=w421, "error code (0)"=1) -> ("error out"=w428:errorcluster)  [unwired: 6 in]
            n156 = Merge Errors(w429, w428) -> (w430:errorcluster)
          }
        }
        n157 = call-dynamic "Delacor_lib_QMH_Error Handler - Message Handling Loop.vi"("error in"=w171, "Message Queue in"=w170) -> ("dup error in"=w172:errorcluster)  [unwired: 8 in, 1 out]
      }
      n158 = call <vilib>:"Set Helper Loop Period.vi"("Period (ms)"=25, "Helper Loop Periodic Timing in"=w21) -> ("Helper Loop Periodic Timing out"=w22:refnum<class "Helper Loop Periodic Timing.lvclass">)  [unwired: 13 in]
      n159 = while "DQMH_HELPER_LOOP" {
        shift-right: [w43] -> w19
        shift-left: w22 -> [w35]
        shift-right: [w41] -> w24
        shift-left: w23 -> [w42]
        tunnel: w27 -> [w38]
        shift-right: [w33] -> _
        shift-left: w18 -> [w34]
        stop <- w40 stop-if-true
        w37 = "Continuous Execution"  # DQMH_HELPER_LOOP_NAME
        # "Continuous Execution"
        n160 = call <vilib>:"Get Timeout.vi"("Helper Loop Periodic Timing"=w35) -> ("Timeout (ms)"=w36:i32)  [unwired: 12 in, 2 out]
        n161 = event "DQMH_HELPER_EVENT_STRUCTURE" shown="[0] Timeout" {
          selector: w42 -> [_ _ _ _]
          dyn-events: [_ _ _ _] -> w41
          timeout: w36 -> [_ _ _ _]
          tunnel: w35 -> [w60 w80 w87 w97]
          tunnel: [w59 w80 w87 w97] -> w43
          tunnel: [_ TRUE _ _] -> w40
          tunnel: [w58 errorcluster {"status"=FALSE, "code"=0, "source"=""} ("error constant") w92 _] -> w39
          tunnel: w38 -> [w57 _ w88 _]
          tunnel: w34 -> [w48 w77 w86 w96]
          tunnel: [w47 w77 w84 w95] -> w33
          event Timeout {
            n162 = event-data() -> ("Time"=w61:u32)  [unwired: 1 in]
            n163 = Unbundle By Name(w48) -> ("Start Time"=w45:timestamp, "Start -Log"=w56:bool, "Stop -Log"=w55:bool, "Data Logging Time (S)"=w46:dbl)
            n164 = call <vilib>:"Update Last Execution Time-v2.vi"("Time"=w61, "Helper Loop Periodic Timing in"=w60) -> ("Helper Loop Periodic Timing out"=w59:refnum<class "Helper Loop Periodic Timing.lvclass">)  [unwired: 12 in, 1 out]
            n165 = Get Date/Time In Seconds() -> (seconds since 1Jan1904=w51:timestamp)
            n166 = To Double Precision Float(number=w51) -> (double precision float=w50:dbl)
            n167 = Build Array(w56, w55) -> (w54:bool[])
            n168 = To Double Precision Float(number=w45) -> (double precision float=w44:dbl)
            n169 = Search 1D Array(1D array=w54, element=TRUE) -> (index of element=w52:i32)  [unwired: 1 in]
            n170 = Increment(x=w52) -> (x+1=w49:i32)
            n171 = case shown="1" w49 {
              tunnel: [_ w75 _] -> w58
              tunnel: w57 -> [_ w74 _]
              tunnel: w50 -> [_ w73 _]
              tunnel: w48 -> [w62 w70 w76]
              tunnel: [w62 w69 w76] -> w47
              tunnel: w46 -> [_ w71 _]
              tunnel: w44 -> [_ w72 _]
              frame 0, Default {
                # "Both Start and Stop are False"
              }
              frame 1 {
                # "Start Log is true"
                n172 = Subtract(x=w73, y=w72) -> (x-y=w63:dbl)
                n173 = Greater Or Equal?(x=w63, y=w71) -> (x >= y?=w67:bool)
                n174 = Select(t="Close TDMS File", s=w67, f="Write to TDMS File") -> (s? t:f=w65:string)
                n175 = Not(x=w67) -> (.not. x?=w68:bool)
                n176 = Bundle By Name(cluster=w70, "Stop -Log"=w67, "Start -Log"=w68) -> (w69:T14)
                n177 = call-poly <vilib>:"Delacor_lib_QMH_Enqueue Message (poly).vi"("Message Data"=w63, "Message"=w65, "Message Queue in"=w74) -> ("error out"=w75:errorcluster)  [unwired: 7 in, 1 out]
              }
              frame 2 {
                # "Stop Log True"
              }
            }
          }
          event User Event {
            n178 = event-data() -> ()  [unwired: 1 in, 1 out]
          }
          event User Event {
            (unwired) "Start Logging"
            n179 = event-data() -> ("Start Logging"=w90:variant)  [unwired: 1 in, 4 out]
            n180 = Bundle(cluster=T2 {"Start Logging"=variant} ("Start Logging Argument"), "Start Logging"=w90) -> (w89:T2)
            n181 = Get Date/Time In Seconds() -> (seconds since 1Jan1904=w83:timestamp)
            n182 = call-poly <vilib>:"Delacor_lib_QMH_Enqueue Message (poly).vi"("Priority Message? (F)"=TRUE, "Message Data"=w89, "Message"="Create TDMS File", "Message Queue in"=w88) -> ("error out"=w92:errorcluster)  [unwired: 6 in, 1 out]
            n183 = Bundle By Name(cluster=w86, "Stop -Log"=FALSE, "Start -Log"=TRUE, "Start Time"=w83) -> (w84:T14)
          }
          event User Event {
            (unwired) T15 {"Data Logging Duration(Sec)"=0.0} ("Data Logging Duration Argument")
            n184 = event-data() -> ("Data Logging Duration(Sec)"=w94:dbl)  [unwired: 1 in]
            n185 = Bundle By Name(cluster=w96, "Data Logging Time (S)"=w94) -> (w95:T14)
            n186 = Bundle("Data Logging Duration(Sec)"=w94) -> ()  [unwired: 1 in, 1 out]
          }
        }
        n187 = call-dynamic "Delacor_lib_QMH_Error Handler - Helper Loop.vi"("Error Debug"=w37, "error in"=w39, "Message Queue in"=w38) -> ()  [unwired: 7 in, 2 out]
      }
      n188 = call <vilib>:"Stop Helper Loop.vi"("Helper Loop Periodic Timing in"=w19) -> ()  [unwired: 1 out]
      n189 = Unregister For Events(event registration refnum=w24) -> ()  [unwired: 1 in, 1 out]
    }
    frame Error {
      # "Synchronize Caller Events.vi will inform Start Module.vi that the module has launched and will let the code calling Start Module.vi register for broadcasts and would permit the caller receive the broadcast that an error occurred at launch time."
      n190 = call-dynamic "Delacor_lib_QMH_Release Message Queue.vi"("error in"=w438, "Message Queue"=w431) -> ("error out"=w437:errorcluster)  [unwired: 9 in]
      n191 = call "Synchronize Caller Events.vi"("Singleton Module Admin in"=w432) -> ("error out"=w439:errorcluster)  [unwired: 9 in, 1 out]
      n192 = call "Module Name--constant.vi"() -> ("Module Name"=w435:string)  [unwired: 11 in]
      n193 = Format Into String(format string="An error occurred during initialization. %s is no longer running.", w435) -> (resulting string=w433:string)  [unwired: 2 in, 1 out]
      n194 = Merge Errors(w437, w439) -> (w440:errorcluster)
      n195 = call "Error Reported.vi"("Additional Information"=w433, "Error"=w440) -> ()  [unwired: 9 in, 1 out]
    }
  }
  n196 = Merge Errors(w14, w17) -> (w13:errorcluster)
  n197 = call "Close Module.vi"("error in"=w13, "Module Admin in"=w8) -> ("error out"=w15:errorcluster, "External Launch"=w2:bool, "Module Admin out"=w3:refnum<class "Delacor_lib_QMH_Module Admin.lvclass">)  [unwired: 7 in]
  n198 = Unregister For Events(event registration refnum=w7, error in=w15) -> (error out=w12:errorcluster)
  "error out" <- w12
  n199 = case "External Launch?" shown="True" w2 {
    tunnel: w12 -> [_ w441]
    frame False {
    }
    frame True {
      n200 = case shown="No Error" w441 {
        frame No Error {
          n201 = invoke on="Invoke Node" class="VI" method="FP.Close"() -> ()  [unwired: 3 in, 3 out]
        }
        frame Error {
          n202 = invoke on="Invoke Node" class="VI" method="FP.Open"("Activate"=TRUE ("Activate?")) -> ()  [unwired: 4 in, 5 out]
        }
      }
    }
  }
  n203 = local write "Module Admin"(w3) -> ()
  n204 = disable-structure shown="Disabled" {
    frame Disabled {
      n205 = TDMS Set Properties(5:string[] ["t"] ("property names"), 7:string[] ["NI_ExpXDimension"] ("property names"), 10:"Parameters") -> ()  [unwired: 3 in, 4 out]
    }
    frame Enabled {
    }
  }
